vi "getServerNotifications.vi"(8 "error in (no error)":errorcluster, 11 "TcpServerBase in":refnum<class "TcpServerBase.lvclass">) -> (0 "error out":errorcluster, 3 "TcpServerBase out":refnum<class "TcpServerBase.lvclass">)   [LabVIEW 2018, in "TcpServerBase.lvclass"]
doc: "Receives a notification from tcpServerCmd and tcpServerTel.\n\nNOTE: put this VI in preallocated reentrant clone execution."
uses:
  TcpServerBase.lvclass
  TcpServer/TcpServer.lvclass
panel:
  in  "stop":bool
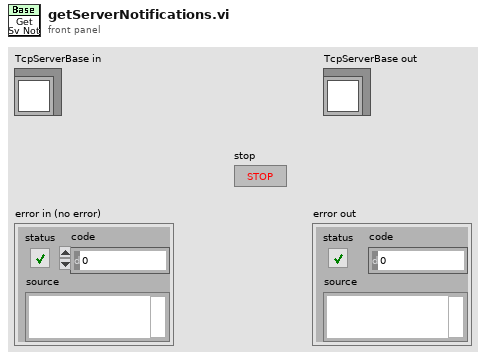
[diagram p1: front panel]
types:
  T1 = cluster{"connectionStatus":bool, "errorSource":string}
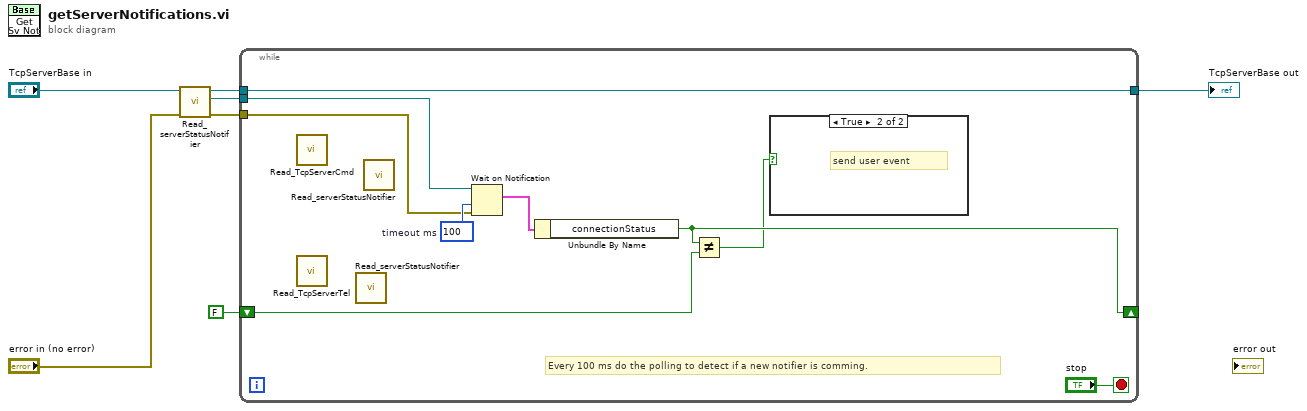
[diagram p0: block diagram]
diagram:
  n1 = call "Read_serverStatusNotifier.vi"("error in (no error)"="error in (no error)", "TcpServerBase in"="TcpServerBase in") -> ("error out"=w4:errorcluster, "serverStatusNotifier"=w6:refnum<notifier>, "TcpServerBase out"=w3:refnum<class "TcpServerBase.lvclass">)  [unwired: 7 in]
  n2 = while {
    tunnel: w6 -> [w15]
    shift-right: [w9] -> _
    shift-left: FALSE -> [w10]
    tunnel: w4 -> [w14]
    tunnel: w3 -> [w13]
    tunnel: [w13] -> w2
    stop <- "stop" stop-if-true
    w16 = 100  # timeout ms
    # "Every 100 ms do the polling to detect if a new notifier is comming."
    n3 = call "Read_TcpServerCmd.vi"() -> ()  [unwired: 9 in, 3 out]
    n4 = call "Read_TcpServerTel.vi"() -> ()  [unwired: 9 in, 3 out]
    n5 = call "Read_serverStatusNotifier.vi"() -> ()  [unwired: 9 in, 3 out]
    n6 = call "Read_serverStatusNotifier.vi"() -> ()  [unwired: 9 in, 3 out]
    n7 = Wait on Notification(notifier=w15, timeout in ms (-1)=w16, error in (no error)=w14) -> (notification=w11:T1)  [unwired: 1 in, 3 out]
    n8 = Unbundle By Name(w11) -> ("connectionStatus"=w9:bool)
    n9 = Not Equal?(x=w9, y=w10) -> (x != y?=w8:bool)
    n10 = case shown="True" w8 {
      frame False {
        # "not send user event"
      }
      frame True {
        # "send user event"
      }
    }
  }
  "TcpServerBase out" <- w2
